vi "ReadControls.vi"(8 "error in (no error)":errorcluster, 11 "Engine in":refnum<class "Engine.lvclass">) -> (0 "error out":errorcluster, 2 "AnyKey?":bool, 3 "Engine out":refnum<class "Engine.lvclass">)   [LabVIEW 2019, in "RT_Game.lvlib" / "Engine.lvclass"]
uses:
  Engine.lvclass
  Engine.lvclass/Engine.ctl
  <vilib>/Utility/error.llb/Error Cluster From Error Code.vi
  <vilib>/rvi/errors/niLvFpgaAdjustHostInterfaceError.vi
  <vilib>/rvi/interface/nirviReadWriteControl/nirviReadWriteControl.xnode
  FPGA_Interface.ctl
  FPGA Bitfiles/myriogameconsole_FPGATarget_Main_ntsPRcBZGxk.lvbitx
  Game/Game.lvclass
  NiFpgaLv.dll
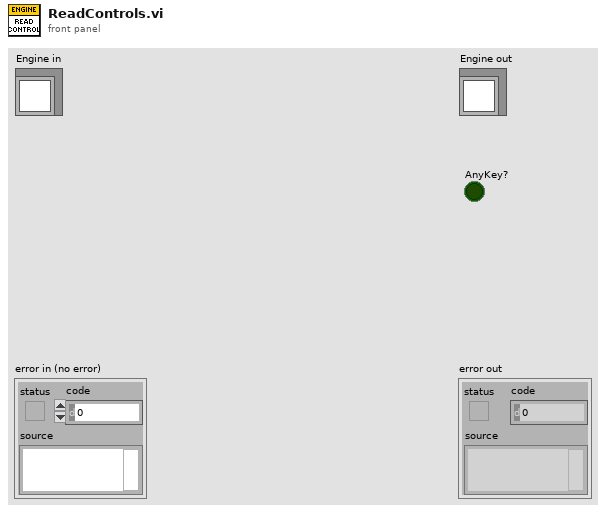
[diagram p1: front panel]
types:
  T1 = typedef "FPGA_Interface.ctl" = refnum<k20>
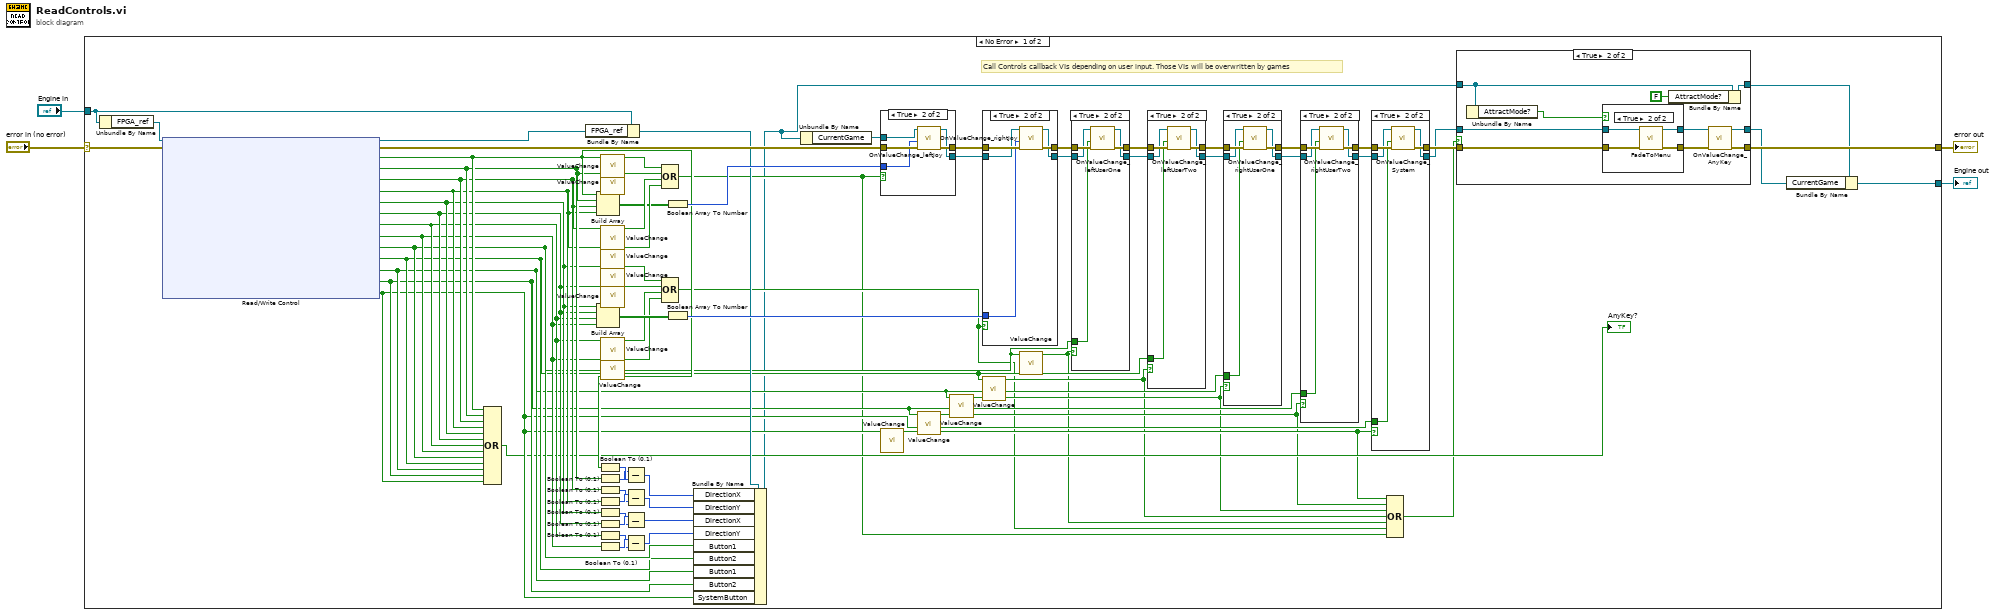
[diagram p0: block diagram]
diagram:
  n1 = case shown="No Error" "error in (no error)" {
    selector: "error in (no error)" -> [w76 w146]
    tunnel: [w18 w146] -> w3
    tunnel: [w52 w145] -> w1
    tunnel: "Engine in" -> [w73 w145]
    frame No Error {
      # "Call Controls callback VIs depending on user input. Those VIs will be overwritten by games"
      n2 = Unbundle By Name(w73) -> ("FPGA_ref"=w74:T1)
      n3 = xnode "Read/Write Control"("FPGA VI Reference In"=w74, "error in"=w76) -> ("FPGA VI Reference Out"=w72:T1, "error out"=w75:errorcluster, "left_left"=w31:bool, "left_right"=w30:bool, "left_up"=w29:bool, "left_down"=w28:bool, "right_left"=w27:bool, "right_right"=w26:bool, "right_up"=w25:bool, "right_down"=w24:bool, "left_1"=w23:bool, "left_2"=w22:bool, "right_1"=w21:bool, "right_2"=w20:bool, "SystemButton"=w19:bool)
      n4 = Compound Arithmetic op=OR(w31, w30, w29, w28, w27, w26, w25, w24, w23, w22, w21, w20, w19) -> (→"AnyKey?":bool)
      n5 = Bundle By Name(cluster=w73, "FPGA_ref"=w72) -> (w32:refnum<class "Engine.lvclass">)
      n6 = Build Array(w31, w30, w29, w28) -> (w67:bool[])
      n7 = Build Array(w27, w26, w25, w24) -> (w64:bool[])
      n8 = Boolean To (0,1)(Boolean=w31) -> (0, 1=w44:i16)
      n9 = Boolean To (0,1)(Boolean=w30) -> (0, 1=w43:i16)
      n10 = Boolean To (0,1)(Boolean=w29) -> (0, 1=w38:i16)
      n11 = Boolean To (0,1)(Boolean=w28) -> (0, 1=w39:i16)
      n12 = Boolean To (0,1)(Boolean=w27) -> (0, 1=w41:i16)
      n13 = Boolean To (0,1)(Boolean=w26) -> (0, 1=w42:i16)
      n14 = Boolean To (0,1)(Boolean=w25) -> (0, 1=w33:i16)
      n15 = Boolean To (0,1)(Boolean=w24) -> (0, 1=w36:i16)
      n16 = call "ValueChange.vi"("left_right"=w31) -> ("Boolean"=w71:bool)  [unwired: 10 in]
      n17 = call "ValueChange.vi"("left_right"=w30) -> ("Boolean"=w70:bool)  [unwired: 10 in]
      n18 = call "ValueChange.vi"("left_right"=w29) -> ("Boolean"=w69:bool)  [unwired: 10 in]
      n19 = call "ValueChange.vi"("left_right"=w28) -> ("Boolean"=w68:bool)  [unwired: 10 in]
      n20 = call "ValueChange.vi"("left_right"=w27) -> ("Boolean"=w60:bool)  [unwired: 10 in]
      n21 = call "ValueChange.vi"("left_right"=w26) -> ("Boolean"=w61:bool)  [unwired: 10 in]
      n22 = call "ValueChange.vi"("left_right"=w25) -> ("Boolean"=w62:bool)  [unwired: 10 in]
      n23 = call "ValueChange.vi"("left_right"=w24) -> ("Boolean"=w63:bool)  [unwired: 10 in]
      n24 = Subtract(x=w43, y=w44) -> (x-y=w40:i16)
      n25 = Subtract(x=w39, y=w38) -> (x-y=w37:i16)
      n26 = Subtract(x=w42, y=w41) -> (x-y=w35:i16)
      n27 = Subtract(x=w36, y=w33) -> (x-y=w34:i16)
      n28 = Compound Arithmetic op=OR(w71, w70, w69, w68) -> (w8:bool)
      n29 = Compound Arithmetic op=OR(w60, w61, w62, w63) -> (w9:bool)
      n30 = Boolean Array To Number(Boolean array=w67) -> (number=w66:u32)
      n31 = Boolean Array To Number(Boolean array=w64) -> (number=w65:u32)
      n32 = Bundle By Name(cluster=w32, "DirectionX"=w40, "DirectionY"=w37, "DirectionX"=w35, "DirectionY"=w34, "Button1"=w23, "Button2"=w22, "Button1"=w21, "Button2"=w20, "SystemButton"=w19) -> (w6:refnum<class "Engine.lvclass">)
      n33 = Unbundle By Name(w6) -> ("CurrentGame"=w51:refnum<class "Game.lvclass">)
      n34 = case shown="True" w8 {
        tunnel: w75 -> [w139 w144]
        tunnel: [w139 w143] -> w59
        tunnel: w66 -> [_ w142]
        tunnel: w51 -> [w138 w141]
        tunnel: [w138 w140] -> w50
        frame False {
        }
        frame True {
          n35 = call-dynamic "OnValueChange_leftJoy.vi"("error in (no error)"=w144, "direction"=w142, "Game in"=w141) -> ("error out"=w143:errorcluster, "Game out"=w140:refnum<class "Game.lvclass">)  [unwired: 7 in]
        }
      }
      n36 = call "ValueChange.vi"("left_right"=w19) -> ("Boolean"=w14:bool)  [unwired: 10 in]
      n37 = call "ValueChange.vi"("left_right"=w20) -> ("Boolean"=w13:bool)  [unwired: 10 in]
      n38 = call "ValueChange.vi"("left_right"=w21) -> ("Boolean"=w12:bool)  [unwired: 10 in]
      n39 = case shown="True" w9 {
        tunnel: w59 -> [w132 w137]
        tunnel: [w132 w136] -> w58
        tunnel: w65 -> [_ w135]
        tunnel: w50 -> [w131 w134]
        tunnel: [w131 w133] -> w49
        frame False {
        }
        frame True {
          n40 = call-dynamic "OnValueChange_rightJoy.vi"("error in (no error)"=w137, "direction"=w135, "Game in"=w134) -> ("error out"=w136:errorcluster, "Game out"=w133:refnum<class "Game.lvclass">)  [unwired: 7 in]
        }
      }
      n41 = call "ValueChange.vi"("left_right"=w22) -> ("Boolean"=w11:bool)  [unwired: 10 in]
      n42 = call "ValueChange.vi"("left_right"=w23) -> ("Boolean"=w10:bool)  [unwired: 10 in]
      n43 = case shown="True" w10 {
        tunnel: w58 -> [w125 w130]
        tunnel: [w125 w129] -> w57
        tunnel: w23 -> [_ w128]
        tunnel: w49 -> [w124 w127]
        tunnel: [w124 w126] -> w48
        frame False {
        }
        frame True {
          n44 = call-dynamic "OnValueChange_leftUserOne.vi"("error in (no error)"=w130, "Value"=w128, "Game in"=w127) -> ("error out"=w129:errorcluster, "Game out"=w126:refnum<class "Game.lvclass">)  [unwired: 7 in]
        }
      }
      n45 = case shown="True" w11 {
        tunnel: w57 -> [w118 w123]
        tunnel: [w118 w122] -> w56
        tunnel: w22 -> [_ w121]
        tunnel: w48 -> [w117 w120]
        tunnel: [w117 w119] -> w47
        frame False {
        }
        frame True {
          n46 = call-dynamic "OnValueChange_leftUserTwo.vi"("error in (no error)"=w123, "Value"=w121, "Game in"=w120) -> ("error out"=w122:errorcluster, "Game out"=w119:refnum<class "Game.lvclass">)  [unwired: 7 in]
        }
      }
      n47 = case shown="True" w12 {
        tunnel: w56 -> [w111 w116]
        tunnel: [w111 w115] -> w55
        tunnel: w21 -> [_ w114]
        tunnel: w47 -> [w110 w113]
        tunnel: [w110 w112] -> w46
        frame False {
        }
        frame True {
          n48 = call-dynamic "OnValueChange_rightUserOne.vi"("error in (no error)"=w116, "Value"=w114, "Game in"=w113) -> ("error out"=w115:errorcluster, "Game out"=w112:refnum<class "Game.lvclass">)  [unwired: 7 in]
        }
      }
      n49 = case shown="True" w13 {
        tunnel: w55 -> [w104 w109]
        tunnel: [w104 w108] -> w54
        tunnel: w20 -> [_ w107]
        tunnel: w46 -> [w103 w106]
        tunnel: [w103 w105] -> w45
        frame False {
        }
        frame True {
          n50 = call-dynamic "OnValueChange_rightUserTwo.vi"("error in (no error)"=w109, "Value"=w107, "Game in"=w106) -> ("error out"=w108:errorcluster, "Game out"=w105:refnum<class "Game.lvclass">)  [unwired: 7 in]
        }
      }
      n51 = case shown="True" w14 {
        tunnel: w54 -> [w97 w102]
        tunnel: [w97 w101] -> w53
        tunnel: w19 -> [_ w100]
        tunnel: [w96 w99] -> w17
        tunnel: w45 -> [w96 w98]
        frame False {
        }
        frame True {
          n52 = call-dynamic "OnValueChange_System.vi"("error in (no error)"=w102, "Value"=w100, "Game in"=w98) -> ("error out"=w101:errorcluster, "Game out"=w99:refnum<class "Game.lvclass">)  [unwired: 7 in]
        }
      }
      n53 = Compound Arithmetic op=OR(w14, w13, w12, w11, w10, w9, w8) -> (w7:bool)
      n54 = case shown="True" w7 {
        tunnel: w53 -> [w78 w89]
        tunnel: [w78 w88] -> w18
        tunnel: w17 -> [w79 w83]
        tunnel: [w79 w87] -> w16
        tunnel: w6 -> [w77 w81]
        tunnel: [w77 w86] -> w5
        frame False {
        }
        frame True {
          n55 = Unbundle By Name(w81) -> ("AttractMode?"=w80:bool)
          n56 = case shown="True" w80 {
            tunnel: w89 -> [w90 w95]
            tunnel: [w90 w94] -> w84
            tunnel: w83 -> [w91 w93]
            tunnel: [w91 w92] -> w82
            frame False {
            }
            frame True {
              n57 = call "FadeToMenu.vi"("error in (no error)"=w95, "Game in"=w93) -> ("error out"=w94:errorcluster, "Game out"=w92:refnum<class "Game.lvclass">)  [unwired: 8 in]
            }
          }
          n58 = Bundle By Name(cluster=w81, "AttractMode?"=FALSE) -> (w86:refnum<class "Engine.lvclass">)
          n59 = call-dynamic "OnValueChange_AnyKey.vi"("error in (no error)"=w84, "Game in"=w82) -> ("error out"=w88:errorcluster, "Game out"=w87:refnum<class "Game.lvclass">)  [unwired: 8 in]
        }
      }
      n60 = Bundle By Name(cluster=w5, "CurrentGame"=w16) -> (w52:refnum<class "Engine.lvclass">)
    }
    frame Error {
    }
  }
  "error out" <- w3
  "Engine out" <- w1
